vi "TrajectoryGenerate_Make_Generic.vi"(7 "Spline Type":T1, 8 "traj_config":T8={"MaxVelocity"=0.0, "Max Acceleration"=0.0, "StartVelocity"=0.0, "End Velocity"=0.0, "Reversed"=FALSE, "DiffDrKineConstntDefined"=FALSE, "CentAcellConstntDefined"=FALSE, "DiffDrVoltConstntDefined"=FALSE, "DIFF_DRIVE_KINE_CONSTRAINT"={"Max Speed (M/S)"=0.0, "DIFF_DRIVE_KINEMATICS"={"TrackWidth_Meters"=0.0}, "Max Accel (M/S2)"=99999.0}, "CENTRIPETAL_ACCEL_CONSTRAINT"={"Max Cent Accel"=0.0}, "SwerveDrKineConstntDefined"=FALSE, "SWERVE_DRIVE_KINE_CONSTRAINT"={"Max Speed (M/S)"=0.0, "SwerveKinematics"={"NumModules"=0, "InverseKinematics"=[], "ForwardKinematics"=[], "Modules"=[], "PrevCoR"={"X"=0.0, "Y"=0.0}}}, "DIFF_DRIVE_VOLTAGE_CONSTRAINT"={"Max Voltage"=0.0, "DIFF_DRIVE_KINEMATICS"={"TrackWidth_Meters"=0.0}, "SIMPLE_MOTOR_FF"={"Ks"=0.0, "Kv"=0.0, "Ka"=0.0}}, "MECANUM_DRIVE_KINE_CONSTRAINT"={"Max Speed (M/S)"=0.0, "MECA_DRIVE_KINEMATICS"={"FrontLeft"={"X"=0.0, "Y"=0.0}, "FrontRight"={"X"=0.0, "Y"=0.0}, "RearLeft"={"X"=0.0, "Y"=0.0}, "RearRight"={"X"=0.0, "Y"=0.0}, "InverseKinematics"=[[0.0, 1.0, -1.0, 0.0], [0.0, 1.0, 1.0, 0.0], [0.0, 1.0, 1.0, 0.0], [0.0, 1.0, -1.0, 0.0]], "ForwardKinematics"=[[0.0, 1.0, -1.0, 0.0], [0.0, 1.0, 1.0, 0.0], [0.0, 1.0, 1.0, 0.0], [0.0, 1.0, -1.0, 0.0]], "PrevCoR"={"X"=0.0, "Y"=0.0}}}, "MecanumDrKineConstntDefined"=FALSE} {"MECANUM_DRIVE_KINE_CONSTRAINT"."MECA_DRIVE_KINEMATICS"."PrevCoR"."Y" format="%14.3f"; "MECANUM_DRIVE_KINE_CONSTRAINT"."MECA_DRIVE_KINEMATICS"."PrevCoR"."X" format="%14.3f"; "MECANUM_DRIVE_KINE_CONSTRAINT"."MECA_DRIVE_KINEMATICS"."RearRight"."Y" format="%14.3f"; "MECANUM_DRIVE_KINE_CONSTRAINT"."MECA_DRIVE_KINEMATICS"."RearRight"."X" format="%14.3f"; "MECANUM_DRIVE_KINE_CONSTRAINT"."MECA_DRIVE_KINEMATICS"."RearLeft"."Y" format="%14.3f"; "MECANUM_DRIVE_KINE_CONSTRAINT"."MECA_DRIVE_KINEMATICS"."RearLeft"."X" format="%14.3f"; "MECANUM_DRIVE_KINE_CONSTRAINT"."MECA_DRIVE_KINEMATICS"."FrontRight"."Y" format="%14.3f"; "MECANUM_DRIVE_KINE_CONSTRAINT"."MECA_DRIVE_KINEMATICS"."FrontRight"."X" format="%14.3f"; "MECANUM_DRIVE_KINE_CONSTRAINT"."MECA_DRIVE_KINEMATICS"."FrontLeft"."Y" format="%14.3f"; "MECANUM_DRIVE_KINE_CONSTRAINT"."MECA_DRIVE_KINEMATICS"."FrontLeft"."X" format="%14.3f"; "MECANUM_DRIVE_KINE_CONSTRAINT"."Max Speed (M/S)" format="%20.4f"; "DIFF_DRIVE_VOLTAGE_CONSTRAINT"."SIMPLE_MOTOR_FF"."Ka" format="%13.4f"; "DIFF_DRIVE_VOLTAGE_CONSTRAINT"."SIMPLE_MOTOR_FF"."Kv" format="%13.4f"; "DIFF_DRIVE_VOLTAGE_CONSTRAINT"."SIMPLE_MOTOR_FF"."Ks" format="%13.4f"; "DIFF_DRIVE_VOLTAGE_CONSTRAINT"."DIFF_DRIVE_KINEMATICS"."TrackWidth_Meters" format="%20.4f"; "DIFF_DRIVE_VOLTAGE_CONSTRAINT"."Max Voltage" format="%20.4f"; "SWERVE_DRIVE_KINE_CONSTRAINT"."SwerveKinematics"."PrevCoR"."Y" format="%14.3f"; "SWERVE_DRIVE_KINE_CONSTRAINT"."SwerveKinematics"."PrevCoR"."X" format="%14.3f"; "SWERVE_DRIVE_KINE_CONSTRAINT"."SwerveKinematics"."Modules"."Y" format="%14.3f"; "SWERVE_DRIVE_KINE_CONSTRAINT"."SwerveKinematics"."Modules"."X" format="%14.3f"; "SWERVE_DRIVE_KINE_CONSTRAINT"."Max Speed (M/S)" format="%20.4f"; "CENTRIPETAL_ACCEL_CONSTRAINT"."Max Cent Accel" format="%20.4f"; "DIFF_DRIVE_KINE_CONSTRAINT"."Max Accel (M/S2)" format="%20.4f"; "DIFF_DRIVE_KINE_CONSTRAINT"."DIFF_DRIVE_KINEMATICS"."TrackWidth_Meters" format="%20.4f"; "DIFF_DRIVE_KINE_CONSTRAINT"."Max Speed (M/S)" format="%20.4f"; "End Velocity" format="%20.4f"; "StartVelocity" format="%20.4f"; "Max Acceleration" format="%20.4f"; "MaxVelocity" format="%20.4f"}, 11 "WeightedWayPoints":T2[](array[typedef]) {"SCALAR" format="%14.3f"; "ROTATION"."SIN" format="%13.4f"; "ROTATION"."COS" format="%13.4f"; "ROTATION"."VALUE" format="%13.4f"; "TRANSLATION"."Y" format="%14.3f"; "TRANSLATION"."X" format="%14.3f"}) -> (0 "error out":errorcluster, 3 "TRAJECTORY":T5 {"States"."POSE"."ROTATION"."SIN" format="%13.4f"; "States"."POSE"."ROTATION"."COS" format="%13.4f"; "States"."POSE"."ROTATION"."VALUE" format="%13.4f"; "States"."POSE"."TRANSLATION"."Y" format="%14.3f"; "States"."POSE"."TRANSLATION"."X" format="%14.3f"; "TotalTImeSecs" format="%20.3f"})   [LabVIEW 2019, in "Trajectory_Library.lvlib"]
doc: "Generates a trajectory from the given waypoints and config. The type of spline used and whether to use weights or auto-calcualte weights is provided as an input. \n\nParameters:\n - Spline Type -- An enumerated value indicating what type of spline to use when creating the trajectory.\n - WeightedWaypoints - The array of waypoints. If weights are not to be used, set the values to zero..\n - Trajectory Config - The configuration for the trajectory.\n\nReturns:\n - Trajectory -- Created trajectory data structure\n - Error Out - Returned error cluster"
uses:
  Trajectory_Library.lvlib
  TRAJ_CONFIG.ctl
  TRAJ_CONSTRAINT_DIIF_DRIVE_KINEMATICS.ctl
  DIFF_DRIVE_KINEMATICS.ctl
  TRAJ_CONSTRAINT_CENTRIPETAL_ACCEL.ctl
  TRAJ_CONSTRAINT_SWERVE_DRIVE_KINEMATICS.ctl
  SWERVE_DRIVE_KINEMATICS.ctl
  <vilib>/Analysis/Matrix/Datatypes/RealMatrix.ctl
  TRANSLATION2D.ctl
  TRAJ_CONSTRAINT_DIIF_DRIVE_VOLTAGE.ctl
  SIMPLE_MOTOR_FF.ctl
  TRAJ_CONSTRAINT_MECA_DRIVE_KINEMATICS.ctl
  MECA_DRIVE_KINEMATICS.ctl
  TRAJECTORY.ctl
  TRAJ_STATE.ctl
  POSE2D.ctl
  ROTATION2D.ctl
  WEIGHTED_WAYPOINT.ctl
  TRAJECTORY_SPLINE_TYPE_ENUM.ctl
  <vilib>/Analysis/Matrix/NI_Matrix.lvlib
panel:
  # "ARRAY OF OTHER\nCONSTRAINTS \nGOES HERE.."
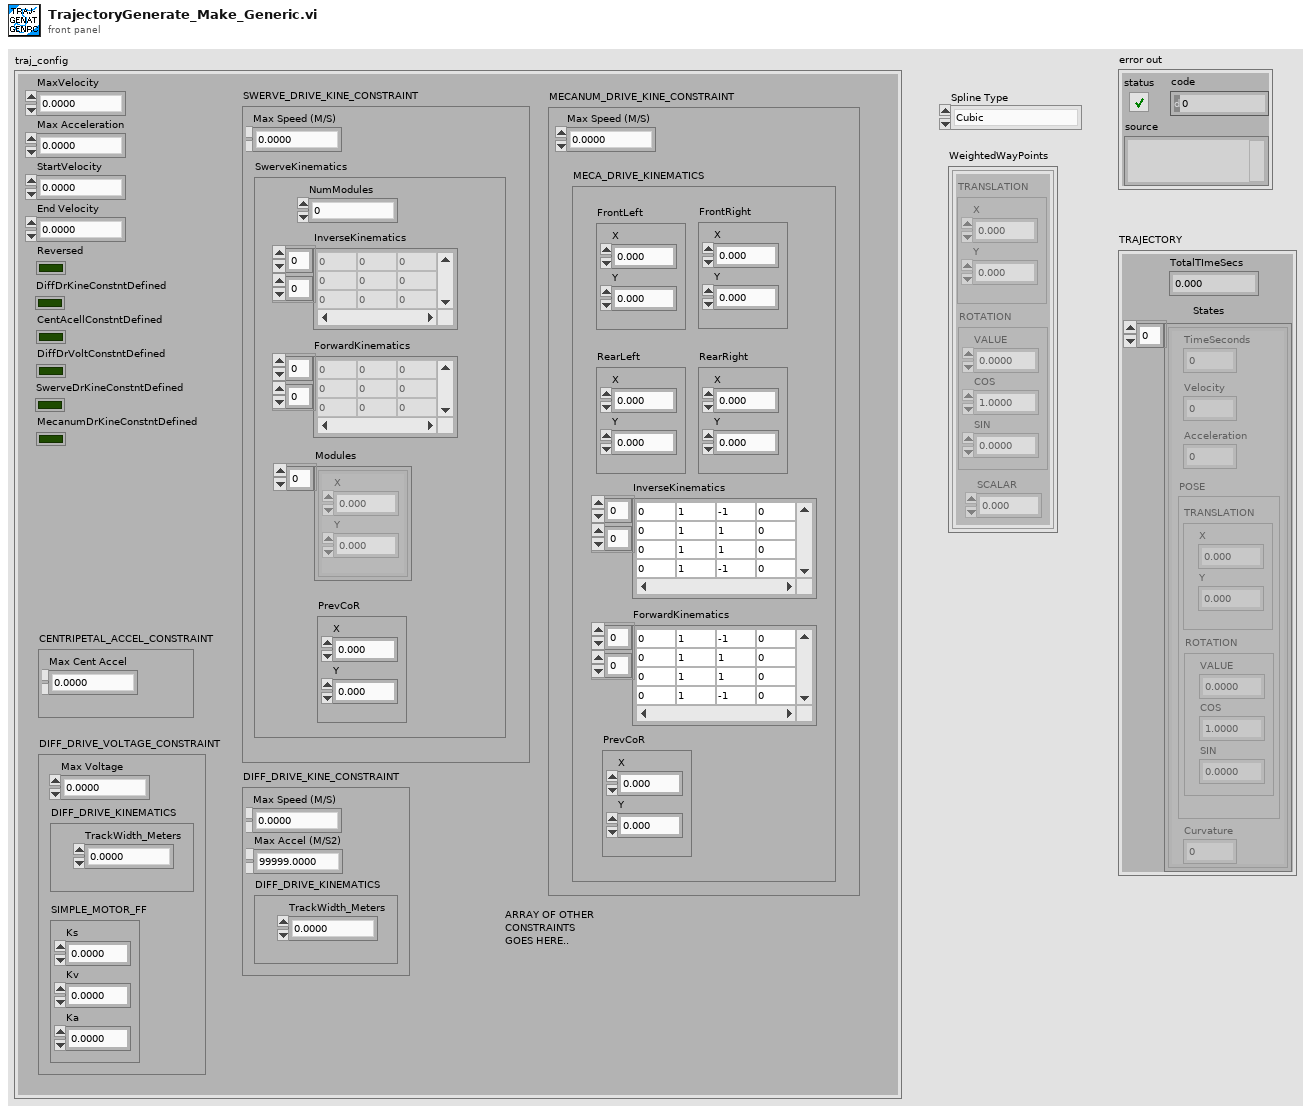
[diagram p1: front panel]
types:
  T1 = typedef "Trajectory_Library.lvlib/TRAJECTORY_SPLINE_TYPE_ENUM.ctl" = enum16{"Cubic", "Cubic With Weights", "Quintic", "Quintic With Weights"}
  T2 = typedef "Trajectory_Library.lvlib/WEIGHTED_WAYPOINT.ctl" = cluster{"TRANSLATION":T3, "ROTATION":T4, "SCALAR":dbl}
  T3 = typedef "Trajectory_Library.lvlib/TRANSLATION2D.ctl" = cluster{"X":dbl, "Y":dbl}
  T4 = typedef "Trajectory_Library.lvlib/ROTATION2D.ctl" = cluster{"VALUE":dbl, "COS":dbl, "SIN":dbl}
  T5 = typedef "Trajectory_Library.lvlib/TRAJECTORY.ctl" = cluster{"TotalTImeSecs":dbl, "States":T6[]}
  T6 = typedef "Trajectory_Library.lvlib/TRAJ_STATE.ctl" = cluster{"TimeSeconds":dbl, "Velocity":dbl, "Acceleration":dbl, "POSE":T7, "Curvature":dbl}
  T7 = typedef "Trajectory_Library.lvlib/POSE2D.ctl" = cluster{"TRANSLATION":T3, "ROTATION":T4}
  T8 = typedef "Trajectory_Library.lvlib/TRAJ_CONFIG.ctl" = cluster{"MaxVelocity":dbl, "Max Acceleration":dbl, "StartVelocity":dbl, "End Velocity":dbl, "Reversed":bool, "DiffDrKineConstntDefined":bool, "CentAcellConstntDefined":bool, "DiffDrVoltConstntDefined":bool, "DIFF_DRIVE_KINE_CONSTRAINT":T9, "CENTRIPETAL_ACCEL_CONSTRAINT":T11, "SwerveDrKineConstntDefined":bool, "SWERVE_DRIVE_KINE_CONSTRAINT":T12, "DIFF_DRIVE_VOLTAGE_CONSTRAINT":T15, "MECANUM_DRIVE_KINE_CONSTRAINT":T17, "MecanumDrKineConstntDefined":bool}
  T9 = typedef "Trajectory_Library.lvlib/TRAJ_CONSTRAINT_DIIF_DRIVE_KINEMATICS.ctl" = cluster{"Max Speed (M/S)":dbl, "DIFF_DRIVE_KINEMATICS":T10, "Max Accel (M/S2)":dbl}
  T10 = typedef "Trajectory_Library.lvlib/DIFF_DRIVE_KINEMATICS.ctl" = cluster{"TrackWidth_Meters":dbl}
  T11 = typedef "Trajectory_Library.lvlib/TRAJ_CONSTRAINT_CENTRIPETAL_ACCEL.ctl" = cluster{"Max Cent Accel":dbl}
  T12 = typedef "Trajectory_Library.lvlib/TRAJ_CONSTRAINT_SWERVE_DRIVE_KINEMATICS.ctl" = cluster{"Max Speed (M/S)":dbl, "SwerveKinematics":T13}
  T13 = typedef "Trajectory_Library.lvlib/SWERVE_DRIVE_KINEMATICS.ctl" = cluster{"NumModules":i32, "InverseKinematics":T14, "ForwardKinematics":T14, "Modules":T3[], "PrevCoR":T3}
  T14 = typedef "NI_Matrix.lvlib/RealMatrix.ctl" = dbl[][]
  T15 = typedef "Trajectory_Library.lvlib/TRAJ_CONSTRAINT_DIIF_DRIVE_VOLTAGE.ctl" = cluster{"Max Voltage":dbl, "DIFF_DRIVE_KINEMATICS":T10, "SIMPLE_MOTOR_FF":T16}
  T16 = typedef "Trajectory_Library.lvlib/SIMPLE_MOTOR_FF.ctl" = cluster{"Ks":dbl, "Kv":dbl, "Ka":dbl}
  T17 = typedef "Trajectory_Library.lvlib/TRAJ_CONSTRAINT_MECA_DRIVE_KINEMATICS.ctl" = cluster{"Max Speed (M/S)":dbl, "MECA_DRIVE_KINEMATICS":T18}
  T18 = typedef "Trajectory_Library.lvlib/MECA_DRIVE_KINEMATICS.ctl" = cluster{"FrontLeft":T3, "FrontRight":T3, "RearLeft":T3, "RearRight":T3, "InverseKinematics":T14, "ForwardKinematics":T14, "PrevCoR":T3}
  T19 = typedef "Trajectory_Library.lvlib/SPLINE_CTRL_VECTOR.ctl" = cluster{"Xs":dbl[], "Ys":dbl[]}
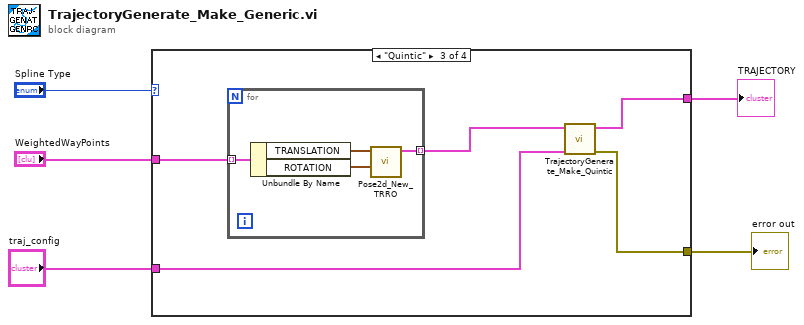
[diagram p0: block diagram]
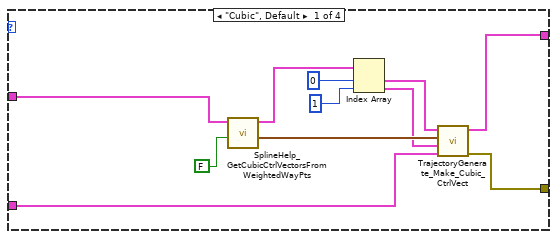
[diagram p2: hidden frame]
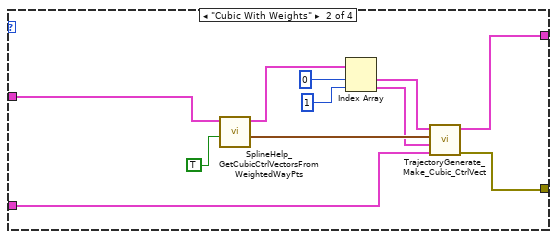
[diagram p3: hidden frame]
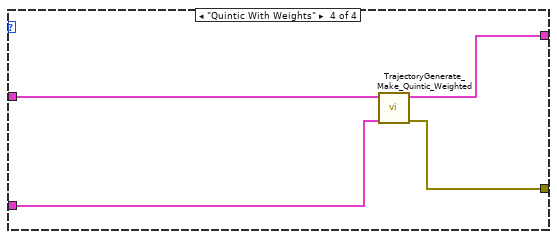
[diagram p4: hidden frame]
diagram:
  n1 = case shown="\"Quintic\"" "Spline Type" {
    tunnel: [w7 w18 w32 w40] -> w4
    tunnel: "traj_config" -> [w8 w20 w30 w37]
    tunnel: "WeightedWayPoints" -> [w9 w19 w29 w38]
    tunnel: [w6 w17 w31 w39] -> w1
    frame "Cubic", Default {
      n2 = call "SplineHelp_GetCubicCtrlVectorsFromWeightedWayPts.vi"("Use Weights"=FALSE, "WeightedWayPoints"=w9) -> ("Interior WAYPOINTS"=w16:T3[], "SplineControlVectors"=w13:T19[])  [unwired: 8 in]
      n3 = Index Array(array=w13, index #1=0 ("index"), index #2=1 ("index")) -> (element #1=w11:T19, element #2=w10:T19)
      n4 = call "TrajectoryGenerate_Make_Cubic_CtrlVect.vi"("traj_config"=w8, "end-Spline_Ctrl_Vector"=w10, "Interior WAYPOINTS"=w16, "initial-Spline_Ctrl_Vector"=w11) -> ("error out"=w6:errorcluster, "TRAJECTORY"=w7:T5)  [unwired: 6 in]
    }
    frame "Cubic With Weights" {
      n5 = call "SplineHelp_GetCubicCtrlVectorsFromWeightedWayPts.vi"("Use Weights"=TRUE, "WeightedWayPoints"=w19) -> ("Interior WAYPOINTS"=w27:T3[], "SplineControlVectors"=w24:T19[])  [unwired: 8 in]
      n6 = Index Array(array=w24, index #1=0 ("index"), index #2=1 ("index")) -> (element #1=w22:T19, element #2=w21:T19)
      n7 = call "TrajectoryGenerate_Make_Cubic_CtrlVect.vi"("traj_config"=w20, "end-Spline_Ctrl_Vector"=w21, "Interior WAYPOINTS"=w27, "initial-Spline_Ctrl_Vector"=w22) -> ("error out"=w17:errorcluster, "TRAJECTORY"=w18:T5)  [unwired: 6 in]
    }
    frame "Quintic" {
      n8 = for {
        tunnel: w29 -> [w36] mode=indexing
        tunnel: [w33] -> w28 mode=indexing
        n9 = Unbundle By Name(w36) -> ("TRANSLATION"=w35:T3, "ROTATION"=w34:T4)
        n10 = call "Pose2d_New_TRRO.vi"("ROTATION"=w34, "TRANSLATION"=w35) -> ("outPOSE"=w33:T7)  [unwired: 9 in]
      }
      n11 = call "TrajectoryGenerate_Make_Quintic.vi"("traj_config"=w30, "waypointPOSE"=w28) -> ("error out"=w31:errorcluster, "TRAJECTORY"=w32:T5)  [unwired: 8 in]
    }
    frame "Quintic With Weights" {
      n12 = call "TrajectoryGenerate_Make_Quintic_Weighted.vi"("traj_config"=w37, "WeightedWaypointPOSE"=w38) -> ("error out"=w39:errorcluster, "TRAJECTORY"=w40:T5)  [unwired: 8 in]
    }
  }
  "TRAJECTORY" <- w4
  "error out" <- w1
